vi "Number Sequence Steps.vi"(0 "Sequence Names":string[][](array[string])) -> (1 "ItemNames Out":string[][](array[string]), 2 "Size":i32)   [LabVIEW 2018]
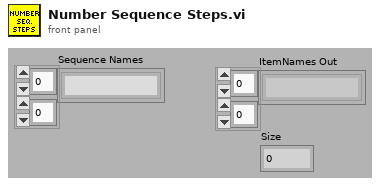
[diagram p1: front panel]
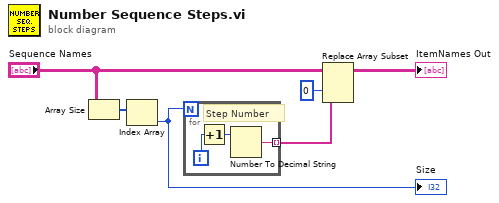
[diagram p0: block diagram]
diagram:
  n1 = Array Size(array="Sequence Names") -> (size(s)=w2:i32[])
  n2 = Index Array(array=w2) -> (element=w1:i32)  [unwired: 1 in]
  "Size" <- w1
  n3 = for {
    N: w1 -> [_]
    tunnel: [w7] -> w5 mode=indexing
    i -> [w9]
    # "Step Number"
    n4 = Increment(x=w9) -> (x+1=w8:i32)
    n5 = Number To Decimal String(number=w8) -> (decimal integer string=w7:string)  [unwired: 1 in]
  }
  n6 = Replace Array Subset(array="Sequence Names", new element=w5, index (col)=0 ("disabled index (col)")) -> (→"ItemNames Out":string[][])  [unwired: 1 in]
